vi "GetIconTemplatePath.vi"() -> (3 "icon template":path)   [LabVIEW 2017, in "MessageGen.lvlib"]
uses:
  <vilib>/addons/InsightCM/MessageBus/CodeGen/MessageGen.lvlib
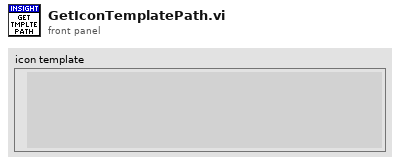
[diagram p1: front panel]
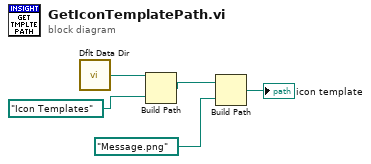
[diagram p0: block diagram]
diagram:
  n1 = call <vilib>:"Dflt Data Dir.vi"() -> ("App:Default Data Directory"=w5:path)
  n2 = Build Path(base path=w5, name or relative path=path "Icon Templates" ("App:Default Data Directory")) -> (appended path=w3:path)
  n3 = Build Path(base path=w3, name or relative path=path "Message.png" ("App:Default Data Directory")) -> (appended path=→"icon template":path)
